vi "Test Process within App Log Error Message.vi"(8 "error in (no error)":errorcluster, 11 "Test Case In":refnum<class "Logger Test.lvclass">) -> (0 "error out":errorcluster, 3 "Test Case Out":refnum<class "Logger Test.lvclass">)   [LabVIEW 2020, in "Logger Test.lvclass"]
uses:
  Logger Test.lvclass
  C:/Program Files (x86)/National Instruments/LabVIEW 2020/vi.lib/Asteme/LUnit/Test Case.lvclass
  Mock Log Handler/Mock Log Handler.lvclass
  C:/Users/anton/Documents/GitHub/Triarc-Framework/source/Framework/Logging/Logging.lvclass
  Framework/Application/Application.lvclass
  C:/Users/anton/Documents/GitHub/Triarc-Framework/source/Framework/Process/Process.lvclass
  Mock Process/Mock Process.lvclass
  Framework/Process/Process.lvclass/Process.ctl
  Framework/Application/Application.lvclass/Application.ctl
  <vilib>/Asteme/LUnit/Test Case.lvclass/Test Case.ctl
  <vilib>/Asteme/LUnit/LUnit Assertion Result.lvclass/LUnit Assertion Result.ctl
  Framework/Application/Private/Add Process to Map.vi
  Framework/Application/Private/Start Idle Processes if Running.vi
  Framework/Process/Protected/Messaging/Enqueue Message.vi
  Framework/Process/Public/Lifecycle/Get Lifecycle State.vi
  Framework/Process/Protected/SubVIs/Set Context.vi
  Framework/Process/Private/SubVIs/Wait for finish.vi
  Framework/Process/Private/SubVIs/Set Lifecycle State.vi
  <vilib>/Asteme/LUnit/Palette/Pass.vi
  <vilib>/Asteme/LUnit/Palette/Fail.vi
  <vilib>/Asteme/LUnit/Variant to string.vi
  <vilib>/Asteme/LUnit/Set Assertion Type.vi
  Framework/Process/Public/Lifecycle/Leave Process Loop.vi
  <vilib>/Asteme/LUnit/Add test result.vi
  <vilib>/Asteme/LUnit/LUnit Write Passed.vi
  <vilib>/Asteme/LUnit/LUnit Get Test Case.vi
  <vilib>/Asteme/LUnit/Assertion Result/LUnit Get Test Name.vi
  <vilib>/Asteme/LUnit/LUnit Write Message.vi
  <vilib>/Asteme/LUnit/LUnit Write Description.vi
  <vilib>/Asteme/LUnit/LUnit Write Assertion Type.vi
  <vilib>/Asteme/LUnit/Read Test Case Name.vi
  <vilib>/Utility/error.llb/Error Cluster From Error Code.vi
  Framework/Application/Private/Update Context for Owned Processes.vi
  <vilib>/Utility/Data Type/Get Type Information.vi
  <vilib>/Utility/LVClass/Get LV Class Name.vi
  <vilib>/Asteme/LUnit/LUnit Assertion Result.lvclass
  Framework/Process/Process.lvclass
  Framework/Logging/Logging.lvclass
  <vilib>/Asteme/LUnit/Test Case.lvclass
  Support/Framework Test Support.lvlib
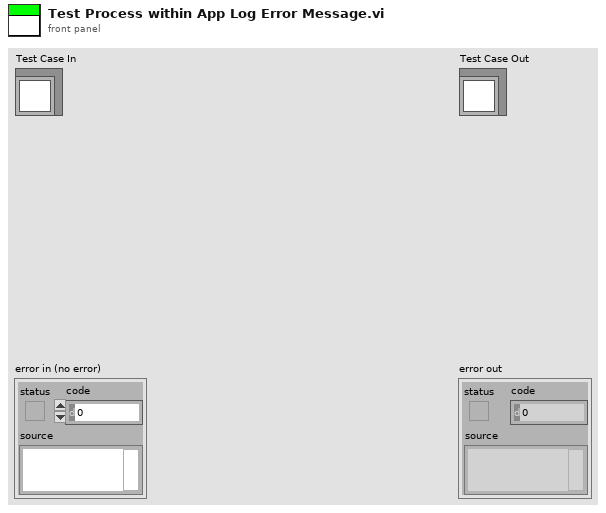
[diagram p1: front panel]
types:
  T1 = typedef "Mock Log Handler.lvclass/Log Entry.ctl" = cluster{"Level":string, "Source":string, "Message":string}
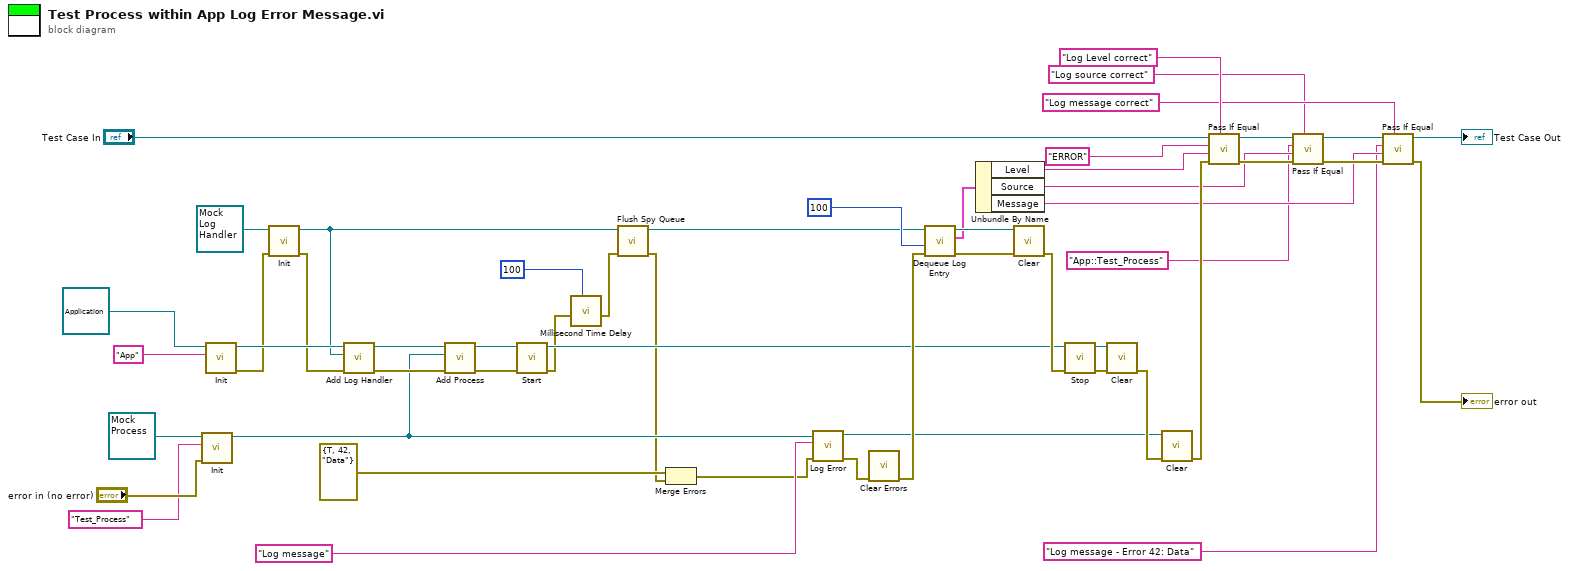
[diagram p0: block diagram]
diagram:
  n1 = call-dynamic "Init.vi"("error in (no error)"="error in (no error)", "Name"="Test_Process", "Mock Process In"=refnum<class "Mock Process.lvclass"> refnum) -> ("Mock Process Out"=w3:refnum<class "Mock Process.lvclass">)  [unwired: 7 in, 1 out]
  n2 = call-dynamic "Init.vi"("Name"="App", "Process In"=refnum<class "Application.lvclass"> refnum ("Application.lvclass")) -> ("error out"=w46:errorcluster, "Process Out"=w49:refnum<class "Application.lvclass">)  [unwired: 8 in]
  n3 = call-dynamic "Init.vi"("error in (no error)"=w46, "Mock Log Handler In"=refnum<class "Mock Log Handler.lvclass"> refnum ("Mock Log Handler.lvclass")) -> ("error out"=w45:errorcluster, "Mock Log Handler Out"=w9:refnum<class "Mock Log Handler.lvclass">)  [unwired: 8 in]
  n4 = call "Add Log Handler.vi"("error in (no error)"=w45, "Log Handler"=w9, "Process In"=w49) -> ("error out"=w19:errorcluster, "Process Out"=w18:refnum<class "Application.lvclass">)  [unwired: 7 in]
  n5 = call "Add Process.vi"("error in (no error)"=w19, "Process"=w3, "Rig In"=w18) -> ("error out"=w15:errorcluster, "Rig Out"=w4:refnum<class "Application.lvclass">)  [unwired: 7 in]
  n6 = call "Start.vi"("error in (no error)"=w15, "Process In"=w4) -> ("error out"=w7:errorcluster, "Process Out"=w11:refnum<class "Application.lvclass">)  [unwired: 8 in]
  n7 = call "Millisecond Time Delay.vi"("milliseconds to wait"=u32 100, "error in (no error)"=w7) -> ("error out"=w6:errorcluster)  [unwired: 7 in]
  n8 = call "Flush Spy Queue.vi"("error in (no error)"=w6, "Mock Log Handler in"=w9) -> ("error out"=w1:errorcluster, "Mock Log Handler out"=w8:refnum<class "Mock Log Handler.lvclass">)  [unwired: 7 in, 1 out]
  n9 = Merge Errors(errorcluster {"status"=TRUE, "code"=42, "source"="Data"} ("error in (no error)"), w1) -> (w2:errorcluster)
  n10 = call "Log Error.vi"("error in (no error)"=w2, "Message"="Log message", "Logging In"=w3) -> ("error out"=w25:errorcluster, "Logging Out"=w12:refnum<class "Mock Process.lvclass">)  [unwired: 7 in]
  n11 = call <vilib>:"Clear Errors.vi"("error in (no error)"=w25) -> ("error out"=w24:errorcluster)  [unwired: 5 in, 1 out]
  n12 = call "Dequeue Log Entry.vi"("error in (no error)"=w24, "timeout in ms (-1)"=100, "Mock Log Handler in"=w8) -> ("error out"=w43:errorcluster, "Entry"=w40:T1, "Mock Log Handler out"=w44:refnum<class "Mock Log Handler.lvclass">)  [unwired: 5 in, 1 out]
  n13 = Unbundle By Name(w40) -> ("Level"=w39:string, "Source"=w29:string, "Message"=w28:string)
  n14 = call-dynamic "Clear.vi"("error in (no error)"=w43, "Mock Log Handler In"=w44) -> ("error out"=w41:errorcluster)  [unwired: 9 in]
  n15 = call "Stop.vi"("error in (no error)"=w41, "Process In"=w11) -> ("error out"=w14:errorcluster, "Process Out"=w13:refnum<class "Application.lvclass">)  [unwired: 7 in, 1 out]
  n16 = call-dynamic "Clear.vi"("error in (no error)"=w14, "Application In"=w13) -> ("error out"=w48:errorcluster)  [unwired: 9 in]
  n17 = call-dynamic "Clear.vi"("error in (no error)"=w48, "Mock Process In"=w12) -> ("error out"=w33:errorcluster)  [unwired: 9 in]
  n18 = call <vilib>:"Pass If Equal.vi"("Description"="Log Level correct", "error in (no error)"=w33, "Actual"=w39, "Expected"="ERROR", "Test Case In"="Test Case In") -> ("error out"=w35:errorcluster, "Test Case Out"=w51:refnum<class "Logger Test.lvclass">)  [unwired: 5 in]
  n19 = call <vilib>:"Pass If Equal.vi"("Description"="Log source correct", "error in (no error)"=w35, "Actual"=w29, "Expected"="App::Test_Process" ("Name"), "Test Case In"=w51) -> ("error out"=w34:errorcluster, "Test Case Out"=w37:refnum<class "Logger Test.lvclass">)  [unwired: 5 in]
  n20 = call <vilib>:"Pass If Equal.vi"("Description"="Log message correct", "error in (no error)"=w34, "Actual"=w28, "Expected"="Log message - Error 42: Data" ("Message"), "Test Case In"=w37) -> ("error out"=→"error out":errorcluster, "Test Case Out"=→"Test Case Out":refnum<class "Logger Test.lvclass">)  [unwired: 5 in]
